vi "FPGA_BaselineSampling.vi"() -> ()   [LabVIEW 2021]
uses:
  <vilib>/rvi/eio/common/nirviEmuTemplateMethod_errors.vi
  <vilib>/rvi/Emulation/niFpgaSctlEmulationGetInTimedLoop.vi
  <vilib>/rvi/Emulation/niFpgaProcessEmulError.vi
  <vilib>/eio/EIONode/EIONode.xnode
panel:
  in  "CurrentSampleRate us":u32
  in  "DCVolt V":fxp<+/-,32,16>
  out "Baseline":fxp<+/-,32,16> format="%.6g"
  out "Done?":bool
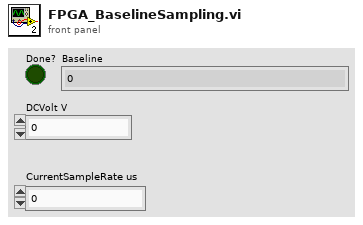
[diagram p1: front panel]
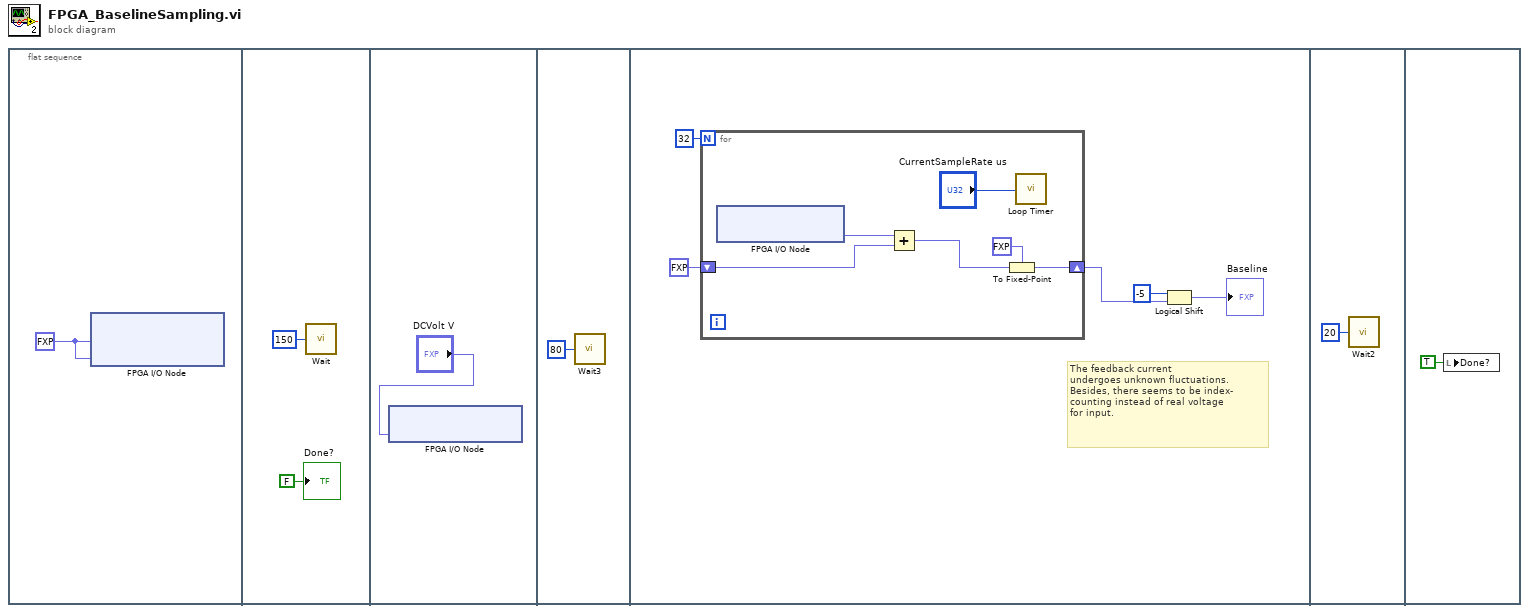
[diagram p0: block diagram]
diagram:
  n1 = flat-sequence {
    frame #0 {
      w1 = fxp<+/-,20,5> 0.0 ("Connector0/AO0")
      n2 = xnode "FPGA I/O Node"("Connector0/AO0"=w1, "Connector0/AO1"=w1) -> ()  [unwired: 2 in, 2 out]
    }
    frame #1 {
      n3 = call "Wait"("Count(mSec)"=u32 150) -> ()  [unwired: 1 out]
      "Done?" <- FALSE
    }
    frame #2 {
      n4 = xnode "FPGA I/O Node"("Connector0/AO3"="DCVolt V") -> ()  [unwired: 1 in, 1 out]
    }
    frame #3 {
      n5 = call "Wait3"("Count(mSec)"=u32 80) -> ()  [unwired: 1 out]
    }
    frame #4 {
      # "The feedback current \nundergoes unknown fluctuations. \nBesides, there seems to be index-\ncounting instead of real voltage \nfor input."
      n6 = for {
        N: 32 -> [_]
        shift-right: [w11] -> w6
        shift-left: fxp<+/-,32,16> 0.0 -> [w14]
        n7 = xnode "FPGA I/O Node"() -> ("Connector0/AI3"=w16:fxp<+/-,27,5>)  [unwired: 1 in, 1 out]
        n8 = Add(x=w16, y=w14) -> (x+y=w12:fxp<+/-,39,17>)
        n9 = To Fixed-Point(fixed-point type=fxp<+/-,32,16> 0.0, number=w12) -> (fixed-point=w11:fxp<+/-,32,16>)
        n10 = call "Loop Timer"("Count(uSec)"="CurrentSampleRate us") -> ()  [unwired: 1 out]
      }
      n11 = Logical Shift(y=i16 -5, x=w6) -> (x << y=→"Baseline":fxp<+/-,32,16>)
    }
    frame #5 {
      n12 = call "Wait2"("Count(mSec)"=u32 20) -> ()  [unwired: 1 out]
    }
    frame #6 {
      n13 = local write "Done?"(TRUE) -> ()
    }
  }
